vi "SaveDialog.vi"(8 "error in":errorcluster, 11 "state in":T1) -> (0 "error out":errorcluster, 1 "new":bool, 3 "state out":T1)   [LabVIEW 2014, in "CI Project Builder.lvlib"]
doc: "This VI ask if you want to save the changes. Depending on the response and the validity of the ccurrent path, it will save the configuration or display the save as dialog."
uses:
  CI Project Builder.lvlib
  Controls/StateCluster.ctl
  <vilib>/ni/Configuration Framework/Node/NodeRef.ctl
  <vilib>/ni/Configuration Framework/Node/NISE_CEF_Node.lvclass
  <vilib>/ni/Configuration Framework/Node/StandardEvents.ctl
  <vilib>/ni/Configuration Framework/Node/UserEventRef.ctl
  <vilib>/ni/Configuration Framework/Controls/EventCluster.ctl
  <vilib>/ni/Configuration Framework/Node/NodeChangeEvent.ctl
  <vilib>/ni/Configuration Framework/Node/CacheState.ctl
  <vilib>/ni/Configuration Framework/Node/RefreshUIEvent.ctl
  <vilib>/ni/Configuration Framework/Node/StopEvent.ctl
  <vilib>/ni/Configuration Framework/glyph manager/glyph manager.ctl
  <vilib>/picture/picture.llb/imagedata.ctl
  <vilib>/ni/Configuration Framework/NISE_CEF_TreeControl.lvlib
  <vilib>/ni/Configuration Framework/glyph manager/glyph manager.lvlib
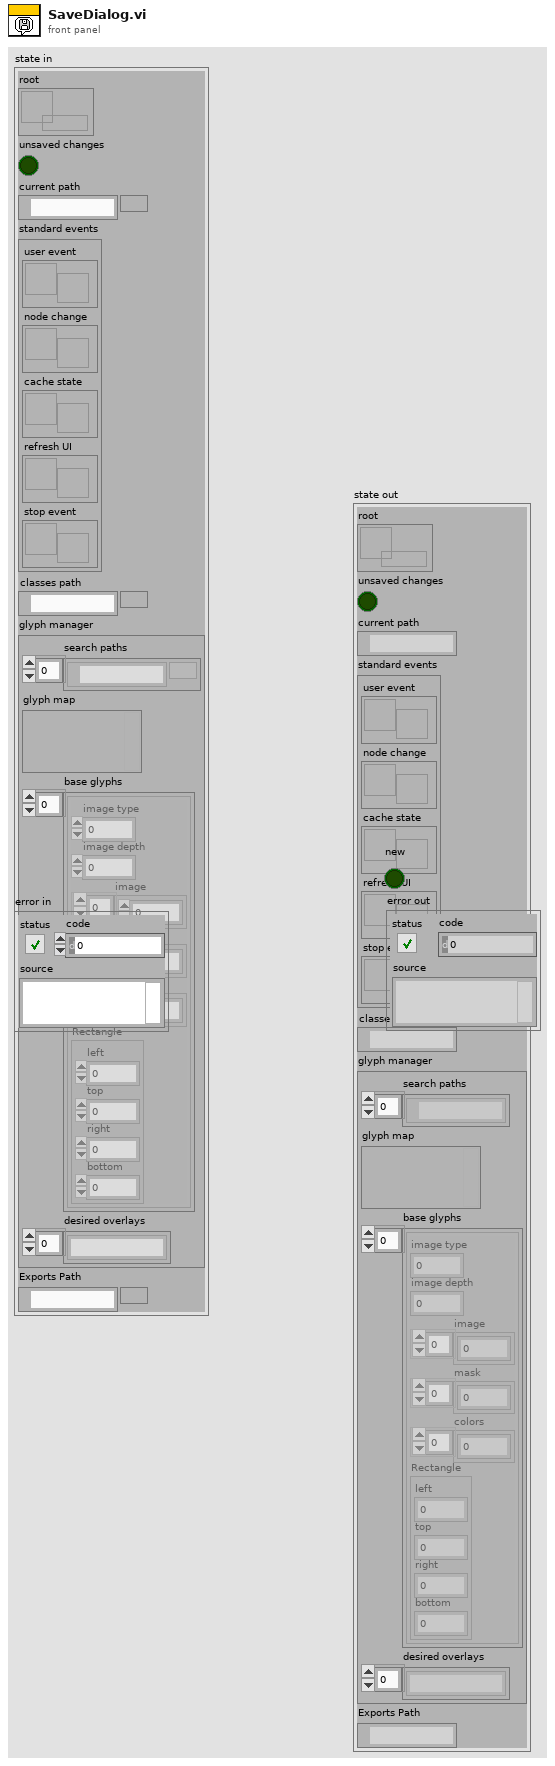
[diagram p1: front panel]
types:
  T1 = typedef "CI Project Builder.lvlib/StateCluster.ctl" = cluster{"root":T2, "unsaved changes":bool, "current path":path, "standard events":T3, "classes path":path, "glyph manager":T9, "Exports Path":path}
  T2 = typedef "NISE_CEF_Node.lvclass/NodeRef.ctl" = refnum<data-value>
  T3 = typedef "NISE_CEF_Node.lvclass/StandardEvents.ctl" = cluster{"user event":T4, "node change":T5, "cache state":T6, "refresh UI":T7, "stop event":T8}
  T4 = typedef "NISE_CEF_Node.lvclass/UserEventRef.ctl" = refnum<user-event>
  T5 = typedef "NISE_CEF_Node.lvclass/NodeChangeEvent.ctl" = refnum<user-event>
  T6 = typedef "NISE_CEF_Node.lvclass/CacheState.ctl" = refnum<user-event>
  T7 = typedef "NISE_CEF_Node.lvclass/RefreshUIEvent.ctl" = refnum<user-event>
  T8 = typedef "NISE_CEF_Node.lvclass/StopEvent.ctl" = refnum<user-event>
  T9 = typedef "glyph manager.lvlib/glyph manager.ctl" = cluster{"search paths":path[], "glyph map":variant, "base glyphs":T10[], "desired overlays":string[]}
  T10 = typedef "imagedata.ctl" = cluster{"image type":i32, "image depth":i32, "image":u8[], "mask":u8[], "colors":u32[], "Rectangle":cluster{"left":i16, "top":i16, "right":i16, "bottom":i16}}
  T11 = enum16{"Left Button", "Center Button", "Right Button", "Window Close"}
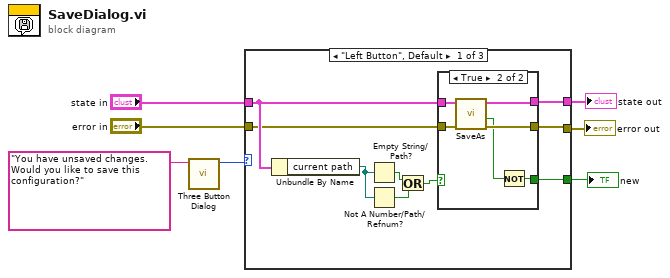
[diagram p0: block diagram]
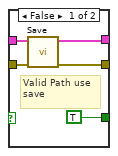
[diagram p2: hidden frame]
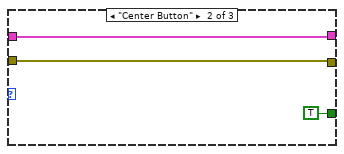
[diagram p3: hidden frame]
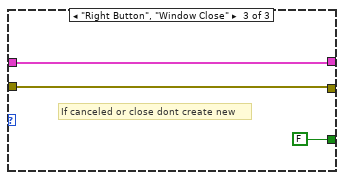
[diagram p4: hidden frame]
diagram:
  n1 = call <vilib>:"Three Button Dialog.vi"("message"="You have unsaved changes.  Would you like to save this configuration?") -> ("Which Button?"=w2:T11)  [unwired: 10 in]
  n2 = case shown="\"Left Button\", Default" w2 {
    tunnel: "state in" -> [w12 w29 w32]
    tunnel: [w11 w29 w32] -> w6
    tunnel: "error in" -> [w9 w28 w31]
    tunnel: [w10 w28 w31] -> w4
    tunnel: [w8 TRUE ("New") FALSE ("New")] -> w1
    frame "Left Button", Default {
      n3 = Unbundle By Name(w12) -> ("current path"=w16:path)
      n4 = Empty String/Path?(string/path=w16) -> (empty?=w14:bool)
      n5 = Not A Number/Path/Refnum?(number/path/refnum=w16) -> (NaN/Path/Refnum?=w13:bool)
      n6 = Or(x=w14, y=w13) -> (x .or. y?=w15:bool)
      n7 = case shown="True" w15 {
        tunnel: w12 -> [w21 w25]
        tunnel: [w20 w24] -> w11
        tunnel: [w19 w26] -> w10
        tunnel: w9 -> [w18 w27]
        tunnel: [TRUE w22] -> w8
        frame False {
          # "Valid Path use save"
          n8 = call "Save.vi"("error in"=w18, "state in"=w21) -> ("error out"=w19:errorcluster, "state out"=w20:T1)  [unwired: 8 in]
        }
        frame True {
          n9 = call "SaveAs.vi"("error in"=w27, "state in"=w25) -> ("error out"=w26:errorcluster, "canceled?"=w23:bool, "state out"=w24:T1)  [unwired: 7 in]
          n10 = Not(x=w23) -> (.not. x?=w22:bool)
        }
      }
    }
    frame "Center Button" {
    }
    frame "Right Button", "Window Close" {
      # "If canceled or close dont create new"
    }
  }
  "state out" <- w6
  "error out" <- w4
  "new" <- w1
